vi "OvrUndrUncert.vi"(6 "StepType":string="_Mag_Step", 7 "Uncert":dbl[][](array[numeric])=[[0.0534457534335421, 0.0596075409674542, 0.0535426680294633, 0.055531987476819866, 0.027916874763925, 0.0300704926380767, 0.0302070361703252, 0.029398134524108967, 0.000210912280974162, 0.0109916584184162], [0.00933227717971764, 0.00609266004408703, 0.008635546341995, 0.008020161188599889, 0.00220129779270583, 0.000447009650582177, 0.000439432672177323, 0.00102924670515511, 0.0, 0.0], [0.00686922407124757, 0.00816016263064548, 0.00252054990386226, 0.005849978868585103, 0.0019279076368534, 0.00329811738218323, 0.00269722918721619, 0.0026410847354176067, 0.0, 0.0], [0.0533186541568546, 0.06008465410288, 0.0538055032227791, 0.055736270494171236, 0.0279918350096046, 0.0301924165653997, 0.0304759612805319, 0.029553404285178733, 0.000233982204691462, 0.0118907125758634], [0.00894311614752633, 0.00648655975890336, 0.0101544881556265, 0.008528054687352063, 0.00189568340081593, 0.000749779537500331, 0.000567248416478003, 0.0010709037849314213, 0.0, 0.0], [0.00695427751824175, 0.0106022352906189, 0.000778626415725707, 0.006111713074862119, 0.00252192526445507, 0.00370913040594196, 0.00342947431774132, 0.0032201766627127835, 0.0, 0.0]], 9 "Limits":dbl[][](array[numeric]), 11 "OvrUndr":dbl[][][](array[numeric])=[[[5.589160017980474, 6.202935187769419, 6.261733208094874, 5.4912209769255735, 5.589161707344972, 6.2029551231392706, 6.261747037530138, 5.491120362323346], [4.572949105620367, 2.0676450625898064, 1.1050117426049793, 4.492817162939127, 4.572950487827704, 2.06765170771309, 1.1050141830935536, 4.492734841900911], [6.250901716245702, 6.12234551147489, 6.422040147832781, 6.094835436401712, 6.2509478685481055, 6.122411699051734, 6.422087384744991, 6.094787216264381], [3.3658701549015175, 3.296647583101864, 1.1333012025587215, 2.0316118121338955, 3.3658950061412862, 3.296683222566312, 1.133309538484409, 2.0315957387548007]], [[5.602495822485004, 6.4906779148884395, 6.442635198982573, 5.491172020965302, 5.602470106718821, 6.490751963178685, 6.442548550239463, 5.4911167638448894], [4.583860218396818, 1.1454137496861998, 2.147545066327524, 4.4927771080625, 4.58383917822449, 1.1454268170315325, 2.1475161834131473, 4.49273189769127], [5.815256963683828, 6.207365165819063, 6.164976794696922, 6.094859384011162, 5.815248363338124, 6.207425210758137, 6.1648611681851415, 6.094822673380493], [3.1312922112143546, 1.0954173822033686, 2.054992264898974, 2.0316197946703958, 3.131287580258993, 1.095427978369075, 2.0549537227283805, 2.0316075577934978]]]) -> (2 "PFI":string[][][](array[string])=[[["P", "P", "P", "P", "P", "P", "P", "P"], ["P", "P", "P", "P", "P", "P", "P", "P"], ["P", "P", "P", "P", "P", "P", "P", "P"], ["P", "P", "P", "P", "P", "P", "P", "P"]], [["P", "P", "P", "P", "P", "P", "P", "P"], ["P", "P", "P", "P", "P", "P", "P", "P"], ["P", "P", "P", "P", "P", "P", "P", "P"], ["P", "P", "P", "P", "P", "P", "P", "P"]]], 3 "OvrUndr":dbl[][][](array[numeric])=[[[5.598492295160192, 5.589160017980474, 5.579827740800756, 6.2090278478135055, 6.202935187769419, 6.196842527725332, 6.270368754436869, 6.261733208094874, 6.2530976617528795, 5.499241138114173, 5.4912209769255735, 5.483200815736974, 5.591363005137677, 5.589161707344972, 5.586960409552266, 6.2034021327898525, 6.2029551231392706, 6.202508113488689, 6.262186470202315, 6.261747037530138, 6.261307604857961, 5.492149609028501, 5.491120362323346, 5.490091115618191], [4.582281382800085, 4.572949105620367, 4.563616828440649, 2.0737377226338936, 2.0676450625898064, 2.0615524025457193, 1.1136472889469742, 1.1050117426049793, 1.0963761962629843, 4.500837324127726, 4.492817162939127, 4.484797001750527, 4.57515178562041, 4.572950487827704, 4.570749190034999, 2.068098717363672, 2.06765170771309, 2.067204698062508, 1.1054536157657309, 1.1050141830935536, 1.1045747504213763, 4.493764088606066, 4.492734841900911, 4.491705595195756], [6.26023399342542, 6.250901716245702, 6.241569439065984, 6.128438171518977, 6.12234551147489, 6.116252851430803, 6.430675694174775, 6.422040147832781, 6.413404601490786, 6.102855597590311, 6.094835436401712, 6.086815275213112, 6.253149166340811, 6.2509478685481055, 6.2487465707554, 6.122858708702316, 6.122411699051734, 6.121964689401152, 6.422526817417168, 6.422087384744991, 6.421647952072814, 6.095816462969536, 6.094787216264381, 6.093757969559226], [3.375202432081235, 3.3658701549015175, 3.3565378777218, 3.302740243145951, 3.296647583101864, 3.2905549230577766, 1.1419367489007164, 1.1333012025587215, 1.1246656562167265, 2.0396319733224955, 2.0316118121338955, 2.0235916509452956, 3.368096303933992, 3.3658950061412862, 3.3636937083485803, 3.297130232216894, 3.296683222566312, 3.29623621291573, 1.1337489711565862, 1.133309538484409, 1.1328701058122317, 2.0326249854599556, 2.0315957387548007, 2.030566492049646]], [[5.6114389386325305, 5.602495822485004, 5.593552706337477, 6.4971644746473425, 6.4906779148884395, 6.4841913551295365, 6.452789687138199, 6.442635198982573, 6.432480710826947, 5.499700075652654, 5.491172020965302, 5.4826439662779505, 5.604365790119637, 5.602470106718821, 5.600574423318005, 6.491501742716185, 6.490751963178685, 6.4900021836411845, 6.443115798655941, 6.442548550239463, 6.4419813018229855, 5.492187667629821, 5.4911167638448894, 5.490045860059958], [4.592803334544344, 4.583860218396818, 4.574917102249291, 1.1519003094451032, 1.1454137496861998, 1.1389271899272964, 2.1576995544831505, 2.147545066327524, 2.1373905781718974, 4.501305162749851, 4.4927771080625, 4.484249053375148, 4.585734861625306, 4.58383917822449, 4.5819434948236735, 1.146176596569033, 1.1454268170315325, 1.144677037494032, 2.148083431829625, 2.1475161834131473, 2.1469489349966695, 4.4938028014762015, 4.49273189769127, 4.491660993906338], [5.824200079831354, 5.815256963683828, 5.806313847536301, 6.213851725577966, 6.207365165819063, 6.20087860606016, 6.175131282852548, 6.164976794696922, 6.154822306541296, 6.103387438698514, 6.094859384011162, 6.08633132932381, 5.81714404673894, 5.815248363338124, 5.813352679937307, 6.208174990295637, 6.207425210758137, 6.206675431220637, 6.165428416601619, 6.1648611681851415, 6.164293919768664, 6.095893577165425, 6.094822673380493, 6.093751769595562], [3.140235327361881, 3.1312922112143546, 3.1223490950668285, 1.101903941962272, 1.0954173822033686, 1.0889308224444652, 2.0651467530546004, 2.054992264898974, 2.044837776743347, 2.040147849357748, 2.0316197946703958, 2.0230917399830437, 3.133183263659809, 3.131287580258993, 3.1293918968581766, 1.0961777579065755, 1.095427978369075, 1.0946781988315746, 2.0555209711448583, 2.0549537227283805, 2.0543864743119027, 2.032678461578429, 2.0316075577934978, 2.0305366540085665]]] format="%_3g")   [LabVIEW 2014]
panel:
  # "PreOvr"
  # "PreUndr"
  # "PostOvr"
  # "PostUndr"
  # "VA"
  # "VB"
  # "VC"
  # "V+"
  # "IA"
  # "IB"
  # "IC"
  # "I+"
  # "VA+u"
  # "VA"
  # "VA-u"
  # "VBu"
  # "VB"
  # "VB-u"
  # "VCu"
  # "VCB"
  # "VC-u"
  # "V+u"
  # "V+B"
  # "V+-u"
  # "IA+u"
  # "IA"
  # "IA-u"
  # "IBu"
  # "IB"
  # "IB-u"
  # "ICu"
  # "ICB"
  # "IC-u"
  # "I+u"
  # "I+B"
  # "I+-u"
  # "PreOvr"
  # "PreUndr"
  # "PostOvr"
  # "PostUndr"
  # "IA"
  # "VA"
  # "VB"
  # "VC"
  # "V+"
  # "IB"
  # "IC"
  # "I+"
  # "PreOvr"
  # "PreUndr"
  # "PostOvr"
  # "PostUndr"
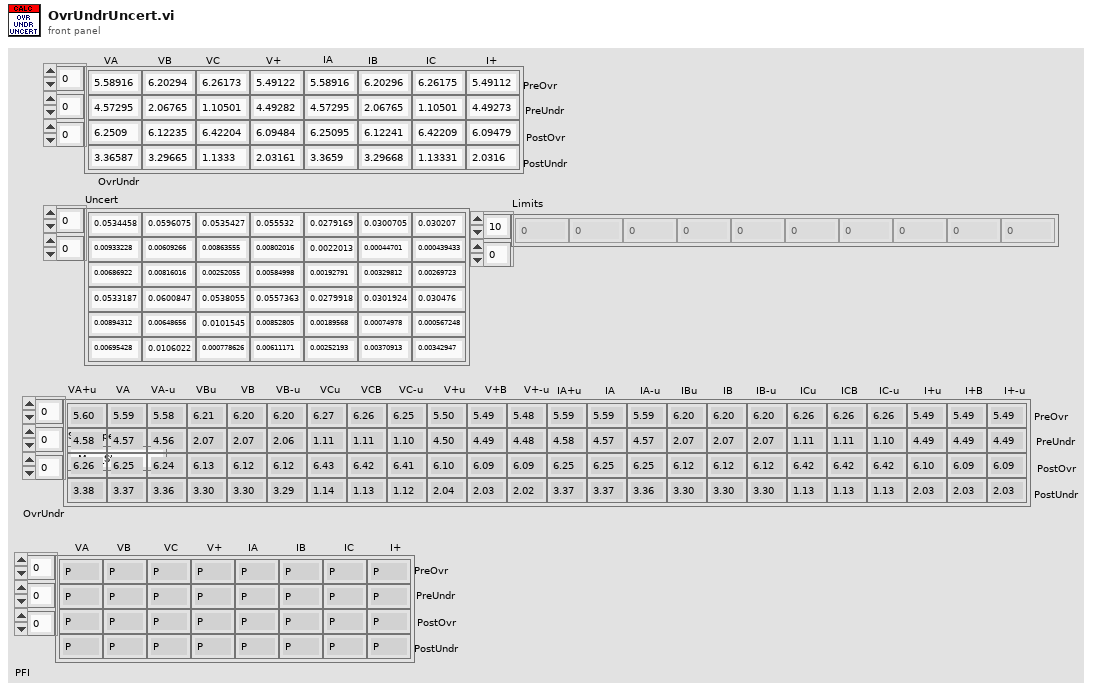
[diagram p1: front panel]
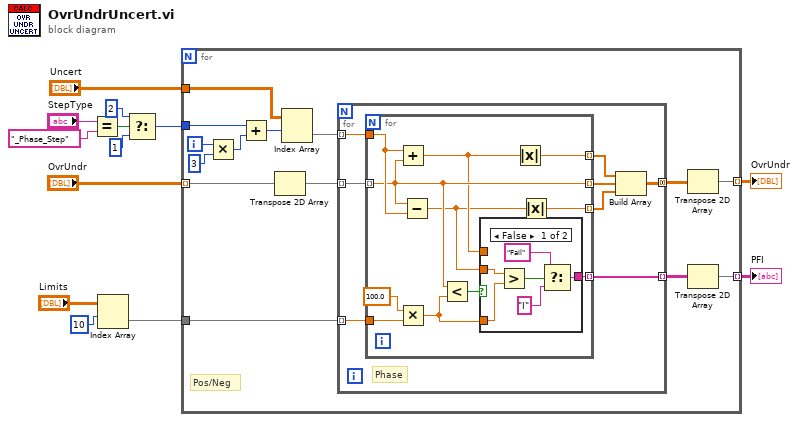
[diagram p0: block diagram]
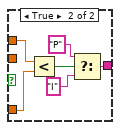
[diagram p2: hidden frame]
diagram:
  n1 = Equal?(x="StepType", y="_Phase_Step") -> (x = y?=w11:bool)
  n2 = Index Array(array="Limits", index (row)=10 ("disabled index (col)")) -> (element=w2:dbl[])  [unwired: 1 in]
  n3 = Select(t=2, s=w11, f=1) -> (s? t:f=w7:i32)
  n4 = for {
    tunnel: "OvrUndr" -> [w21] mode=indexing
    tunnel: w7 -> [w24]
    tunnel: "Uncert" -> [w22]
    tunnel: [w17] -> w5 mode=indexing
    tunnel: [w15] -> w4 mode=indexing
    tunnel: w2 -> [w14]
    i -> [w27]
    # "Pos/Neg"
    n5 = Multiply(x=w27, y=3) -> (x*y=w25:i32)
    n6 = Add(x=w24, y=w25) -> (x+y=w23:i32)
    n7 = Transpose 2D Array(2D array=w21) -> (transposed array=w19:dbl[][])
    n8 = Index Array(array=w22, index (row)=w23) -> (element=w20:dbl[])  [unwired: 1 in]
    n9 = for {
      tunnel: w19 -> [w31] mode=indexing
      tunnel: w20 -> [w35] mode=indexing
      tunnel: [w32] -> w18 mode=concatenating
      tunnel: [w29] -> w16 mode=indexing
      tunnel: w14 -> [w28] mode=indexing
      # "Phase"
      n10 = for {
        tunnel: w35 -> [w46]
        tunnel: [w39] -> w34 mode=indexing
        tunnel: [w40] -> w33 mode=indexing
        tunnel: w31 -> [w45] mode=indexing
        tunnel: [w45] -> w30 mode=indexing
        tunnel: [w41] -> w29 mode=indexing
        tunnel: w28 -> [w38]
        n11 = Add(x=w46, y=w45) -> (x+y=w43:dbl)
        n12 = Multiply(x=100.0 ("y"), y=w38) -> (x*y=w36:dbl)
        n13 = Subtract(x=w45, y=w46) -> (x-y=w42:dbl)
        n14 = Less?(x=w45, y=w36) -> (x < y?=w44:bool)
        n15 = case shown="False" w44 {
          tunnel: w43 -> [_ w58]
          tunnel: w36 -> [w52 w57]
          tunnel: w42 -> [w51 _]
          tunnel: [w47 w53] -> w41
          frame False {
            n16 = Greater?(x=w51, y=w52) -> (0:w50:bool)
            n17 = Select(t="Fail", s=w50, f="I") -> (s? t:f=w47:string)
          }
          frame True {
            n18 = Less?(x=w58, y=w57) -> (x < y?=w56:bool)
            n19 = Select(t="P", s=w56, f="I") -> (s? t:f=w53:string)
          }
        }
        n20 = Absolute Value(x=w43) -> (abs(x)=w40:dbl)
        n21 = Absolute Value(x=w42) -> (abs(x)=w39:dbl)
      }
      n22 = Build Array(w33, w30, w34) -> (w32:dbl[][])
    }
    n23 = Transpose 2D Array(2D array=w18) -> (transposed array=w17:dbl[][])
    n24 = Transpose 2D Array(2D array=w16) -> (transposed array=w15:string[][])
  }
  "OvrUndr" <- w5
  "PFI" <- w4
